vi "uBlaze VIVM.vi"() -> ()   [LabVIEW 2011]
uses:
  <vilib>/Platform/TimedLoop/XDataNode/timing_clust.ctl
  <vilib>/Platform/TimedLoop/XDataNode/nitl_modes.ctl
  <vilib>/Platform/TimedLoop/XDataNode/wakeup.ctl
  <vilib>/rvi/eio/common/nirviEmuTemplateMethod_errors.vi
  Globals.vi
  <vilib>/Platform/TimedLoop/XDataNode/XDataNode.xnode
  <vilib>/eio/EIONode/EIONode.xnode
  <vilib>/Platform/TimedLoop/XDataNode/XDNodeRunTimeDep.lvlib
panel:
  out "Indicator D (+0x001C)":u32 format="%08x"
  out "Indicator C (+0x0018)":u32 format="%08x"
  out "Indicator B (+0x0014)":u32 format="%08x"
  out "Indicator A (+0x0010)":u32 format="%08x"
  out "Control D (+0x000C)":u32 format="%08x"
  out "Control C (+0x0008)":u32 format="%08x"
  out "Control B (+0x0004)":u32 format="%08x"
  out "Control A (+0x0000)":u32 format="%08x"
  out "CS?":bool
  in  "High Address":u32=3225485311 format="%08x"
  in  "Base Address":u32=3225419776 format="%08x"
  out "Write error?":bool
  out "Read Error?":bool
  out "Byte enable?":bool[](array[boolean])
  out "Write data":u32 format="%08x"
  out "Read?":bool
  out "Read data":u32 format="%08x"
  out "Address":u32 format="%08x"
  out "Port0/DIO0":bool
  in  "?":bool
  # "Host Interface"
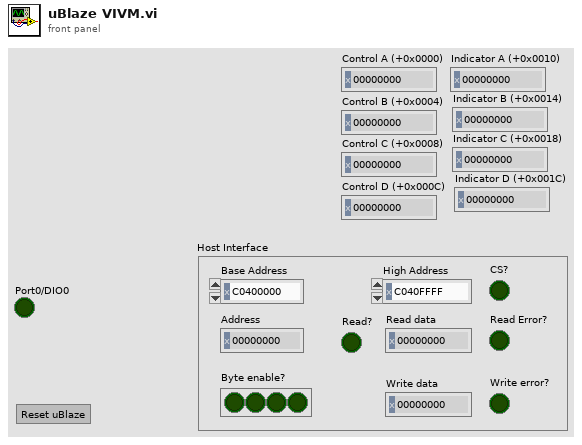
[diagram p1: front panel]
types:
  T1 = typedef "XDNodeRunTimeDep.lvlib/timing_clust.ctl" = cluster{"Expected End [f-1]":u64, "Actual End [f-1]":u64, "Finished Late? [f-1]":bool, "Expected End [i-1]":u64, "Actual End [i-1]":u64, "Finished Late? [i-1]":bool, "Expected Start [i]":u64, "Actual Start [i]":u64, "Expected Start [f]":u64, "Actual Start [f]":u64, "Source Name":string, "Structure Name":string, "Period":i64, "Deadline":i64, "Offset":i64, "Start":i64, "Priority":i32, "Timeout":i32, "Mode":T2, "Wakeup Reason":T3, "Error":errorcluster, "Source Type":string, "Secondary Source Type":string, "Global End Time":u64, "Global Start Time":u64, "Frame Duration":u64, "Iteration Duration":u64, "Assigned CPU":i32, "I/O Scan Engine Mode":u32}
  T2 = typedef "XDNodeRunTimeDep.lvlib/nitl_modes.ctl" = enum32{"No Change", "Process missed periods, maintain original phase", "Discard missed periods, maintain original phase", "Process missed periods, ignore original phase", "Discard missed periods, ignore original phase"}
  T3 = typedef "XDNodeRunTimeDep.lvlib/wakeup.ctl" = enum32{"Normal", "Aborted", "Asynchronous wakeup", "Timing source error", "Timed loop error", "Timeout"}
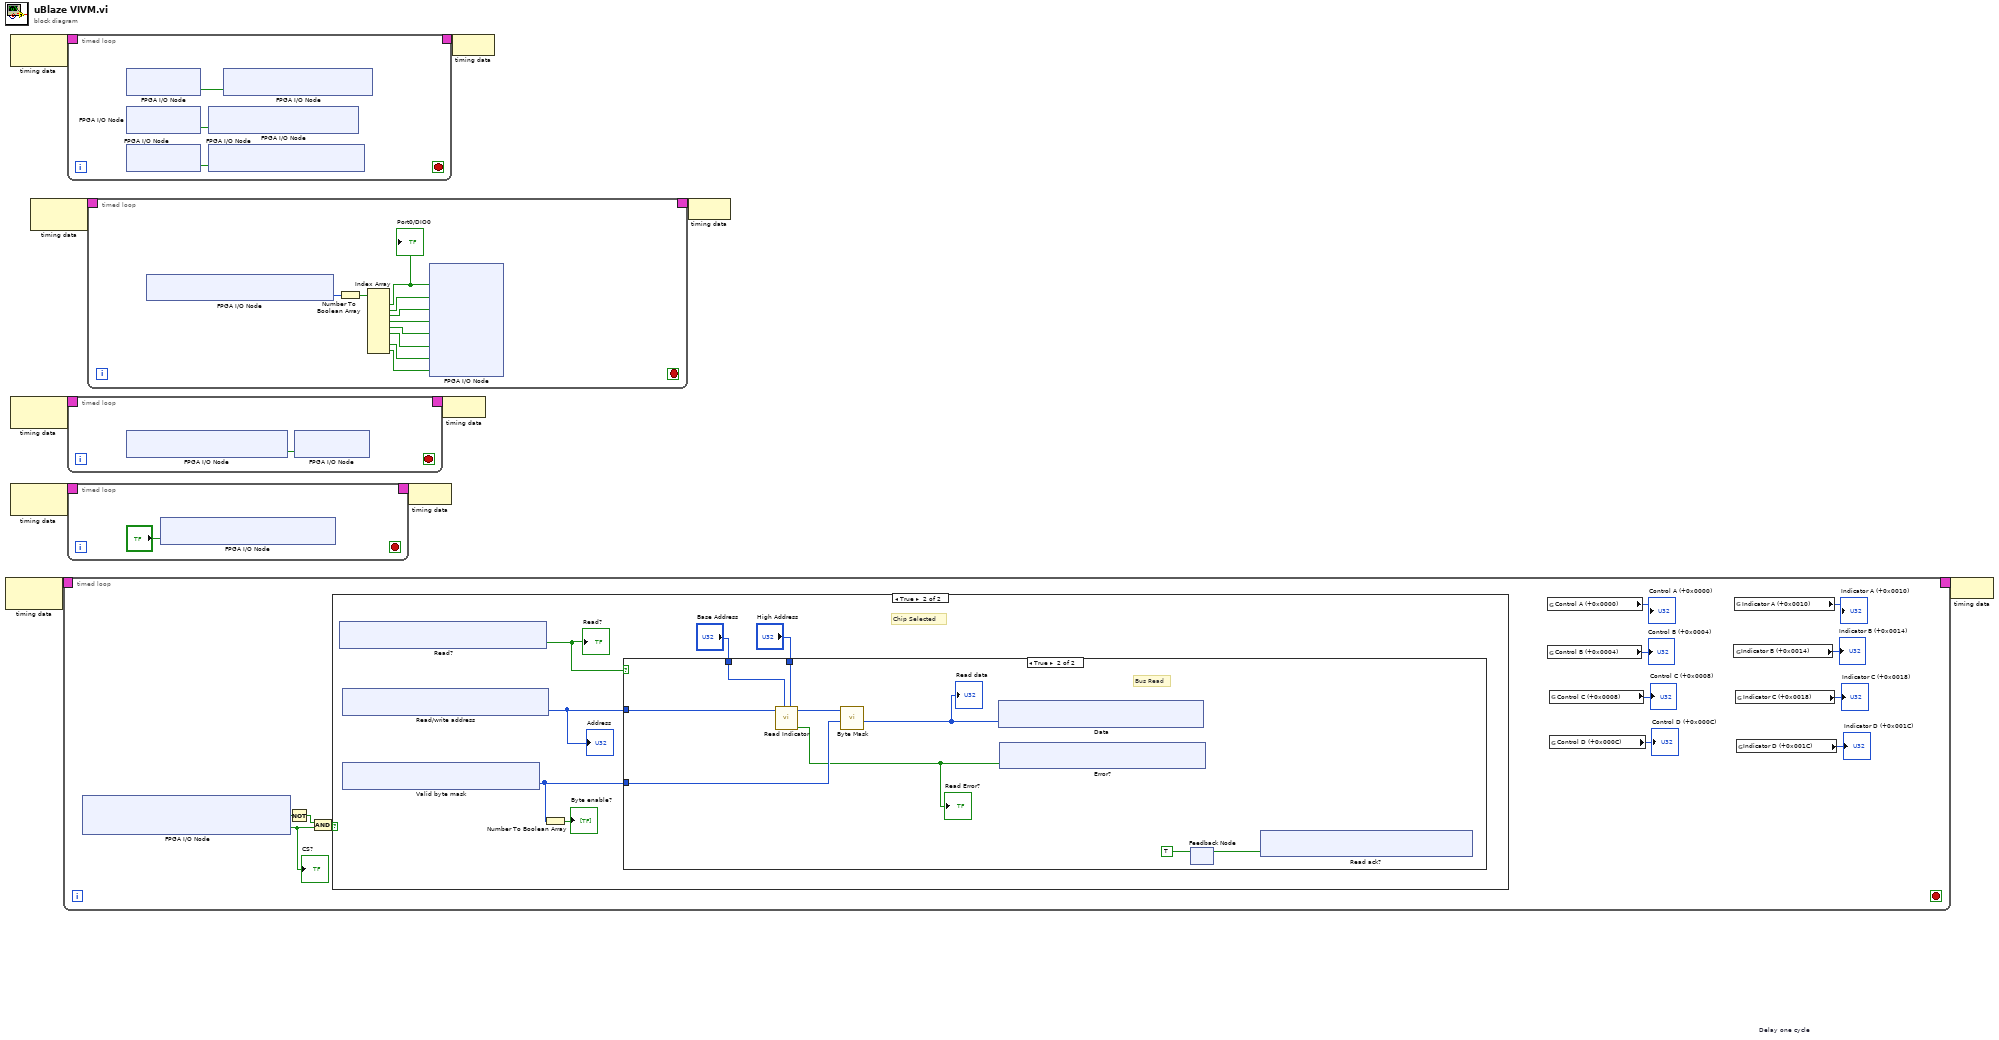
[diagram p0: block diagram]
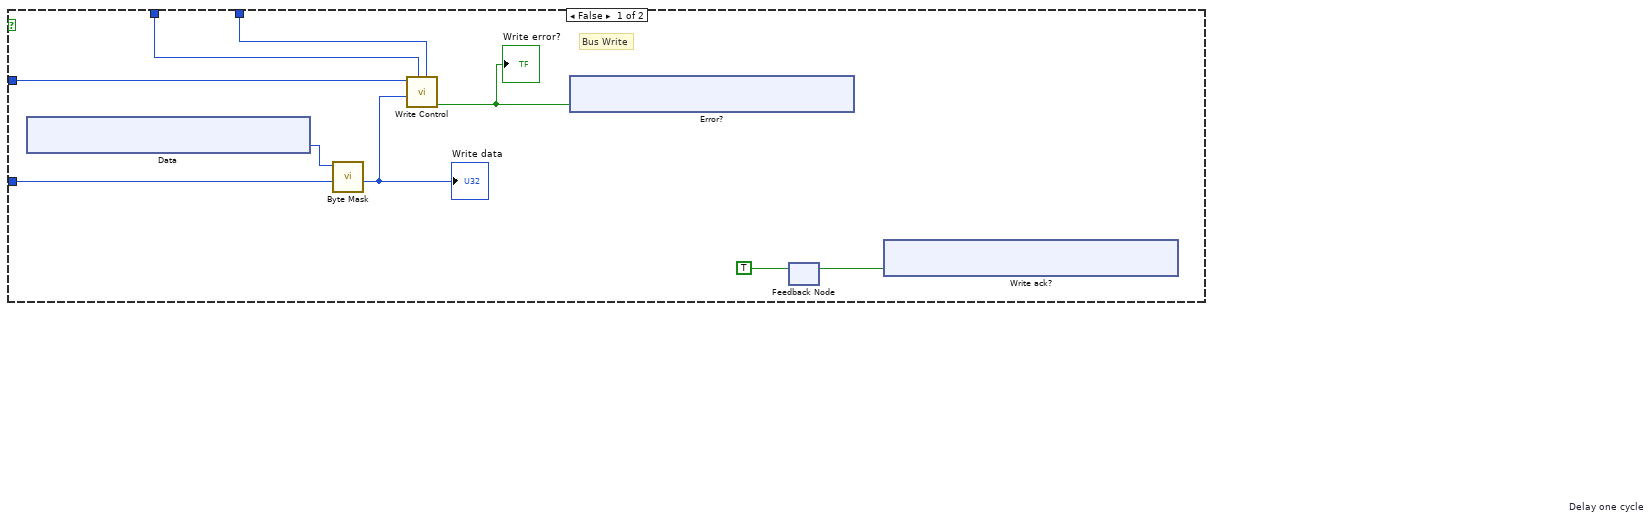
[diagram p3: hidden frame]
diagram:
  n1 = node-c288() -> (w2:T1)  [unwired: 1 in]
  n2 = node-c288() -> (w10:T1)  [unwired: 1 in]
  n3 = node-c288() -> (w8:T1)  [unwired: 1 in]
  n4 = node-c288() -> (w6:T1)  [unwired: 1 in]
  n5 = node-c288() -> (w4:T1)  [unwired: 1 in]
  n6 = timed-loop {
    timing: w2 -> [_]
    timing-out: [_] -> w1
    stop <- _ stop-if-true
    n7 = xnode "FPGA I/O Node"() -> ("myprocessor\\ipic_test_0_ipif_Bus2IP_Reset_pin"=w21:bool, "myprocessor\\ipic_test_0_ipif_Bus2IP_CS_pin"=w19:bool)  [unwired: 2 in, 2 out]
    "CS?" <- w19
    n8 = Not(x=w21) -> (.not. x?=w20:bool)
    n9 = And(x=w20, y=w19) -> (x .and. y?=w22:bool)
    n10 = case shown="True" w22 {
      frame False {
        # "Chip Not Selected/Reset"
      }
      frame True {
        # "Chip Selected"
        n11 = xnode "Read?"() -> ("myprocessor\\ipic_test_0_ipif_Bus2IP_RNW_pin"=w28:bool)  [unwired: 1 in, 1 out]
        "Read?" <- w28
        n12 = xnode "Read/write address"() -> ("myprocessor\\ipic_test_0_ipif_Bus2IP_Addr_pin"=w27:i32)  [unwired: 1 in, 1 out]
        "Address" <- w27
        n13 = xnode "Valid byte mask"() -> ("myprocessor\\ipic_test_0_ipif_Bus2IP_BE_pin"=w25:i8)  [unwired: 1 in, 1 out]
        n14 = Number To Boolean Array(number=w25) -> (Boolean array=→"Byte enable?":bool[])
        n15 = case shown="True" w28 {
          tunnel: w27 -> [w37 w46]
          tunnel: w25 -> [w35 w44]
          tunnel: "Base Address" -> [w32 w40]
          tunnel: "High Address" -> [w31 w41]
          frame False {
            # "Bus Write"
            n16 = xnode "Data"() -> ("myprocessor\\ipic_test_0_ipif_Bus2IP_Data_pin"=w36:i32)  [unwired: 1 in, 1 out]
            n17 = call "Byte Mask.vi"("Byte Mask"=w35, "Data"=w36) -> ("Masked Data"=w34:u32)  [unwired: 9 in]
            "Write data" <- w34
            n18 = call "Write Control.vi"("High Address"=w31, "Base Address"=w32, "Data"=w34, "Address"=w37) -> ("Error"=w33:bool)  [unwired: 7 in]
            "Write error?" <- w33
            n19 = xnode "Error?"("myprocessor\\ipic_test_0_ipif_IP2Bus_Error_pin"=w33) -> ()  [unwired: 1 in, 1 out]
            n20 = feedback-in #1(TRUE ("myprocessor\\ipic_test_0_ipif_IP2Bus_WrAck_pin")) -> ()
            n21 = feedback #1 "Delay one cycle"() -> (w29:bool)  [unwired: 1 in]
            n22 = xnode "Write ack?"("myprocessor\\ipic_test_0_ipif_IP2Bus_WrAck_pin"=w29) -> ()  [unwired: 1 in, 1 out]
          }
          frame True {
            # "Bus Read"
            n23 = call "Read Indicator.vi"("High Address"=w41, "Base Address"=w40, "Address"=w46) -> ("Error"=w42:bool, "Data"=w45:i32)  [unwired: 7 in]
            "Read Error?" <- w42
            n24 = call "Byte Mask.vi"("Byte Mask"=w44, "Data"=w45) -> ("Masked Data"=w43:u32)  [unwired: 9 in]
            "Read data" <- w43
            n25 = xnode "Data"("myprocessor\\ipic_test_0_ipif_IP2Bus_Data_pin"=w43) -> ()  [unwired: 1 in, 1 out]
            n26 = xnode "Error?"("myprocessor\\ipic_test_0_ipif_IP2Bus_Error_pin"=w42) -> ()  [unwired: 1 in, 1 out]
            n27 = feedback-in #2(TRUE ("myprocessor\\ipic_test_0_ipif_IP2Bus_RdAck_pin")) -> ()
            n28 = feedback #2 "Delay one cycle"() -> (w38:bool)  [unwired: 1 in]
            n29 = xnode "Read ack?"("myprocessor\\ipic_test_0_ipif_IP2Bus_RdAck_pin"=w38) -> ()  [unwired: 1 in, 1 out]
          }
        }
      }
    }
    n30 = global read "Globals.vi" "Control A (+0x0000)"() -> (→"Control A (+0x0000)":u32)
    n31 = global read "Globals.vi" "Control B (+0x0004)"() -> (→"Control B (+0x0004)":u32)
    n32 = global read "Globals.vi" "Control C (+0x0008)"() -> (→"Control C (+0x0008)":u32)
    n33 = global read "Globals.vi" "Control D (+0x000C)"() -> (→"Control D (+0x000C)":u32)
    n34 = global read "Globals.vi" "Indicator B (+0x0014)"() -> (→"Indicator B (+0x0014)":u32)
    n35 = global read "Globals.vi" "Indicator A (+0x0010)"() -> (→"Indicator A (+0x0010)":u32)
    n36 = global read "Globals.vi" "Indicator C (+0x0018)"() -> (→"Indicator C (+0x0018)":u32)
    n37 = global read "Globals.vi" "Indicator D (+0x001C)"() -> (→"Indicator D (+0x001C)":u32)
  }
  n38 = timed-loop {
    timing: w10 -> [_]
    timing-out: [_] -> w9
    stop <- _ stop-if-true
    n39 = xnode "FPGA I/O Node"() -> ("Port3/DIO2"=w49:bool)  [unwired: 1 in, 1 out]
    n40 = xnode "FPGA I/O Node"() -> ("Port3/DIO0"=w51:bool)  [unwired: 1 in, 1 out]
    n41 = xnode "FPGA I/O Node"() -> ("Port3/DIO1"=w50:bool)  [unwired: 1 in, 1 out]
    n42 = xnode "FPGA I/O Node"("myprocessor\\mdm_0_TMS_pin"=w51) -> ()  [unwired: 1 in, 1 out]
    n43 = xnode "FPGA I/O Node"("myprocessor\\mdm_0_extTDI_pin"=w50) -> ()  [unwired: 1 in, 1 out]
    n44 = xnode "FPGA I/O Node"("myprocessor\\mdm_0_TCK_pin"=w49) -> ()  [unwired: 1 in, 1 out]
  }
  n45 = timed-loop {
    timing: w8 -> [_]
    timing-out: [_] -> w7
    stop <- _ stop-if-true
    n46 = xnode "FPGA I/O Node"() -> ("myprocessor\\mdm_0_extTDO_pin"=w54:bool)  [unwired: 1 in, 1 out]
    n47 = xnode "FPGA I/O Node"("Port3/DIO3"=w54) -> ()  [unwired: 1 in, 1 out]
  }
  n48 = timed-loop {
    timing: w6 -> [_]
    timing-out: [_] -> w5
    stop <- _ stop-if-true
    n49 = xnode "FPGA I/O Node"("myprocessor\\fpga_0_rst_1_sys_rst_pin"="?") -> ()  [unwired: 1 in, 1 out]
  }
  n50 = timed-loop {
    timing: w4 -> [_]
    timing-out: [_] -> w3
    stop <- _ stop-if-true
    n51 = xnode "FPGA I/O Node"() -> ("myprocessor\\xps_gpio_0_GPIO_IO_O_pin"=w69:i8)  [unwired: 1 in, 1 out]
    n52 = Number To Boolean Array(number=w69) -> (Boolean array=w68:bool[])
    n53 = Index Array(array=w68) -> (element #1=w67:bool, element #2=w66:bool, element #3=w65:bool, element #4=w64:bool, element #5=w63:bool, element #6=w62:bool, element #8=w61:bool, element #9=w60:bool)  [unwired: 9 in, 1 out]
    "Port0/DIO0" <- w67
    n54 = xnode "FPGA I/O Node"("Port0/DIO0"=w67, "Port0/DIO1"=w66, "Port0/DIO2"=w65, "Port0/DIO3"=w64, "Port0/DIO4"=w63, "Port0/DIO5"=w62, "Port0/DIO6"=w61, "Port0/DIO7"=w60) -> ()  [unwired: 8 in, 8 out]
  }
  n55 = node-c288(w5) -> ()
  n56 = node-c288(w7) -> ()
  n57 = node-c288(w9) -> ()
  n58 = node-c288(w3) -> ()
  n59 = node-c288(w1) -> ()
